vi "BLE_Request_ServiceUUIDs.vi"(0 ".NET Refnum in":refnum<k24>, 11 "error in (no error)":errorcluster) -> (4 ".NET Refnum out":refnum<k24>, 8 "ServiceUUIDs":string[](array[string]), 15 "error out":errorcluster)   [LabVIEW 2019]
uses:
  C:/Users/chrismadlax/Desktop/LabVIEW-BLE-Driver/BLELib.dll
  BLELib.dll
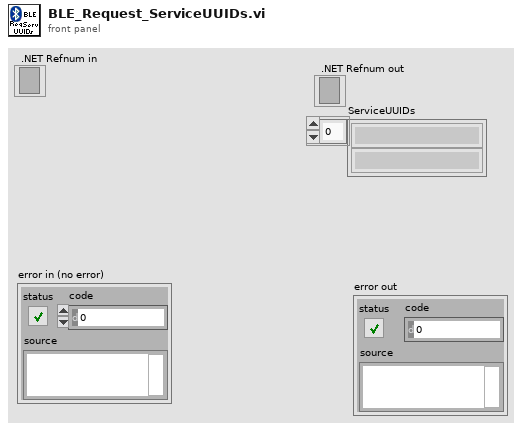
[diagram p1: front panel]
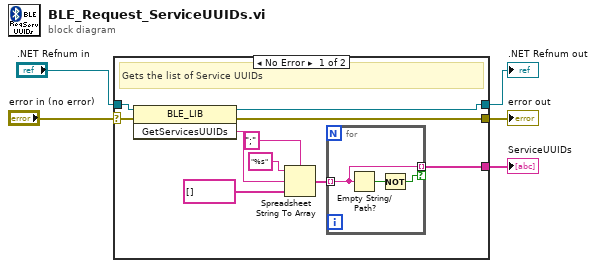
[diagram p0: block diagram]
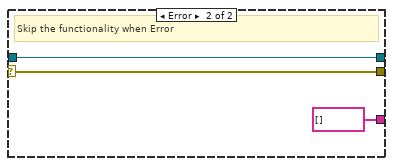
[diagram p2: hidden frame]
diagram:
  n1 = case shown="No Error" "error in (no error)" {
    selector: "error in (no error)" -> [w14 w21]
    tunnel: [w8 w20] -> w5
    tunnel: ".NET Refnum in" -> [w15 w20]
    tunnel: [w6 w21] -> w3
    tunnel: [w9 string[] []] -> w1
    frame No Error {
      # "Gets the list of Service UUIDs"
      n2 = invoke class="BLE_LIB" method="GetServicesUUIDs"(reference=w15, error in=w14) -> (reference out=w8:refnum<k24>, error out=w6:errorcluster, "GetServicesUUIDs"=w7:string)  [unwired: 1 in]
      n3 = Spreadsheet String To Array(delimiter (Tab)=";", format string="%s", spreadsheet string=w7, array type (2D Dbl)=string[] []) -> (array=w13:string[])
      n4 = for {
        tunnel: w13 -> [w18] mode=indexing
        tunnel: [w18] -> w9 mode=indexing if=w16
        n5 = Empty String/Path?(string/path=w18) -> (empty?=w17:bool)
        n6 = Not(x=w17) -> (.not. x?=w16:bool)
      }
    }
    frame Error {
      # "Skip the functionality when Error"
    }
  }
  ".NET Refnum out" <- w5
  "error out" <- w3
  "ServiceUUIDs" <- w1
